vi "indentChildrenXML.vi"(8 "error in (no error)":errorcluster, 9 "childXML":string, 10 "parentElementName":string, 11 "WriteElement in":refnum<class "XMLGenerator.lvclass">) -> (0 "error out":errorcluster, 2 "indentedChildrenXML":string, 3 "WriteElement out":refnum<class "XMLGenerator.lvclass">)   [LabVIEW 2014, in "XML.lvlib" / "XMLGenerator.lvclass"]
doc: "This method indents the XML input depending on the level (first level no indent, second level indent 2 spaces)"
uses:
  <userlib>/Common/XML/XMLGenerator/XMLGenerator.lvclass
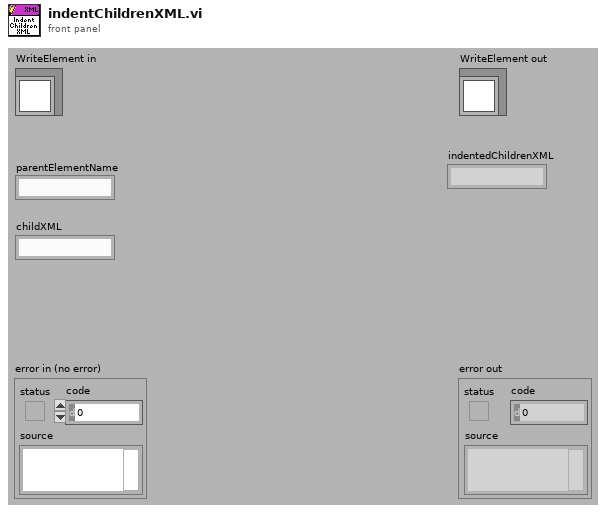
[diagram p1: front panel]
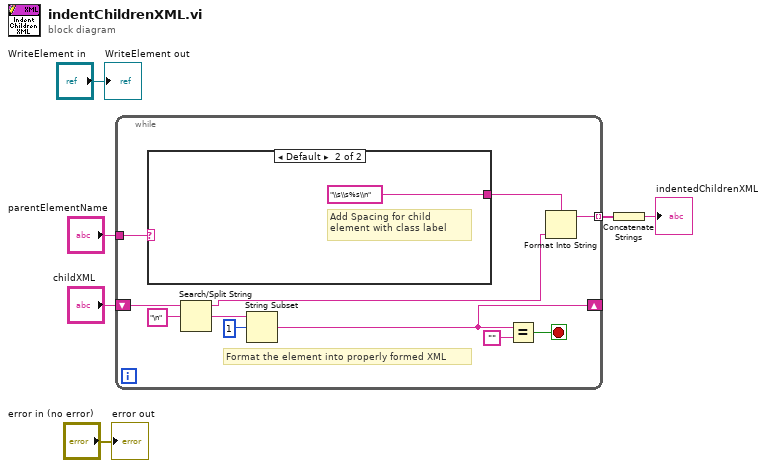
[diagram p0: block diagram]
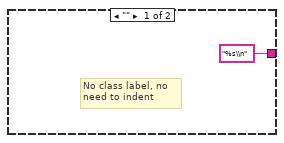
[diagram p2: hidden frame]
diagram:
  n1 = while {
    tunnel: [w7] -> w2 mode=indexing
    shift-right: [w9] -> _
    shift-left: "childXML" -> [w11]
    tunnel: "parentElementName" -> [w8]
    stop <- w16 stop-if-true
    # "Format the element into properly formed XML"
    n2 = case shown="Default" w8 {
      tunnel: ["%s\\n" ("format string") "\\s\\s%s\\n" ("format string")] -> w14
      frame "" {
        # "No class label, no need to indent"
      }
      frame Default {
        # "Add Spacing for child element with class label"
      }
    }
    n3 = Search/Split String(string=w11, search string/char (-)="\n" ("delimiter (Tab)")) -> (substring before match=w10:string, match + rest of string=w13:string)  [unwired: 1 in, 1 out]
    n4 = String Subset(string=w13, offset (0)=1) -> (substring=w9:string)  [unwired: 1 in]
    n5 = Equal?(x=w9, y="") -> (x = y?=w16:bool)
    n6 = Format Into String(format string=w14, w10) -> (resulting string=w7:string)  [unwired: 2 in, 1 out]
  }
  n7 = Concatenate Strings(w2) -> (→"indentedChildrenXML":string)
  "error out" <- "error in (no error)"
  "WriteElement out" <- "WriteElement in"
